vi "SRI8610C-ProcessSRILogFile.vi"(8 "error in":errorcluster) -> (0 "error out":errorcluster, 1 "Butane % Array":string[](array[string]), 2 "GC Full Data Channels":T1[](array[typedef]), 4 "Formatted Data Output":string[][](array[string]), 6 "Raw Data":string)   [LabVIEW 2020, in "SRI8610C-GasChromatograph.lvlib"]
uses:
  SRI8610C-GasChromatograph.lvlib
  Controls/SRI8610C-DataClusterV2.ctl
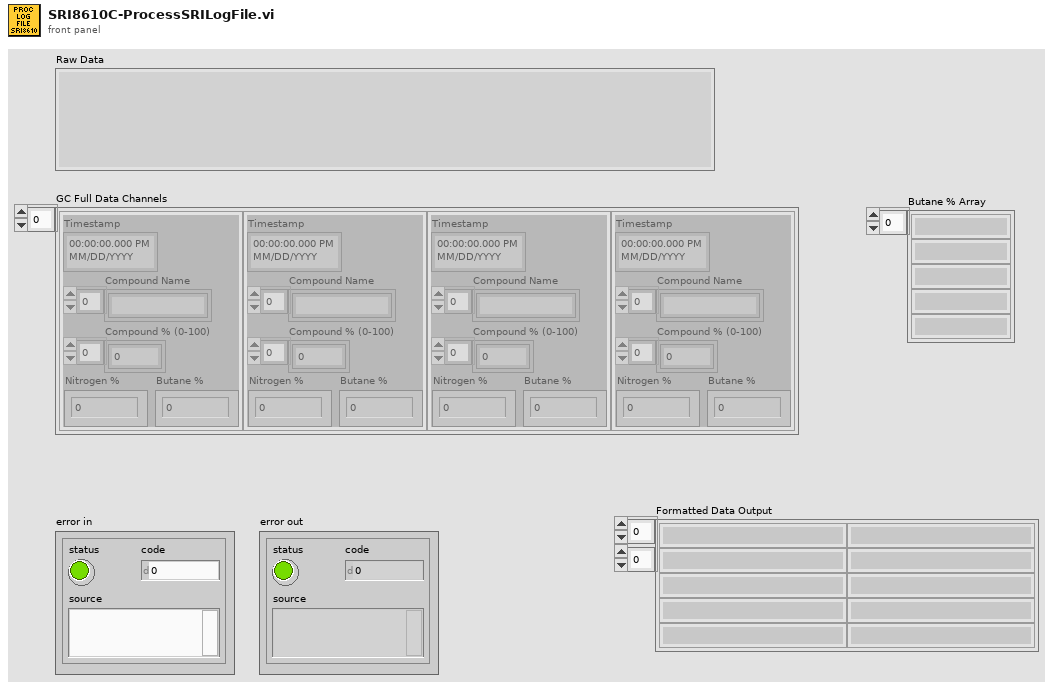
[diagram p1: front panel]
types:
  T1 = typedef "SRI8610C-DataClusterV2.ctl" = cluster{"Timestamp":timestamp, "Compound Name":string[], "Compound % (0-100)":dbl[], "Nitrogen %":dbl, "Butane %":dbl}
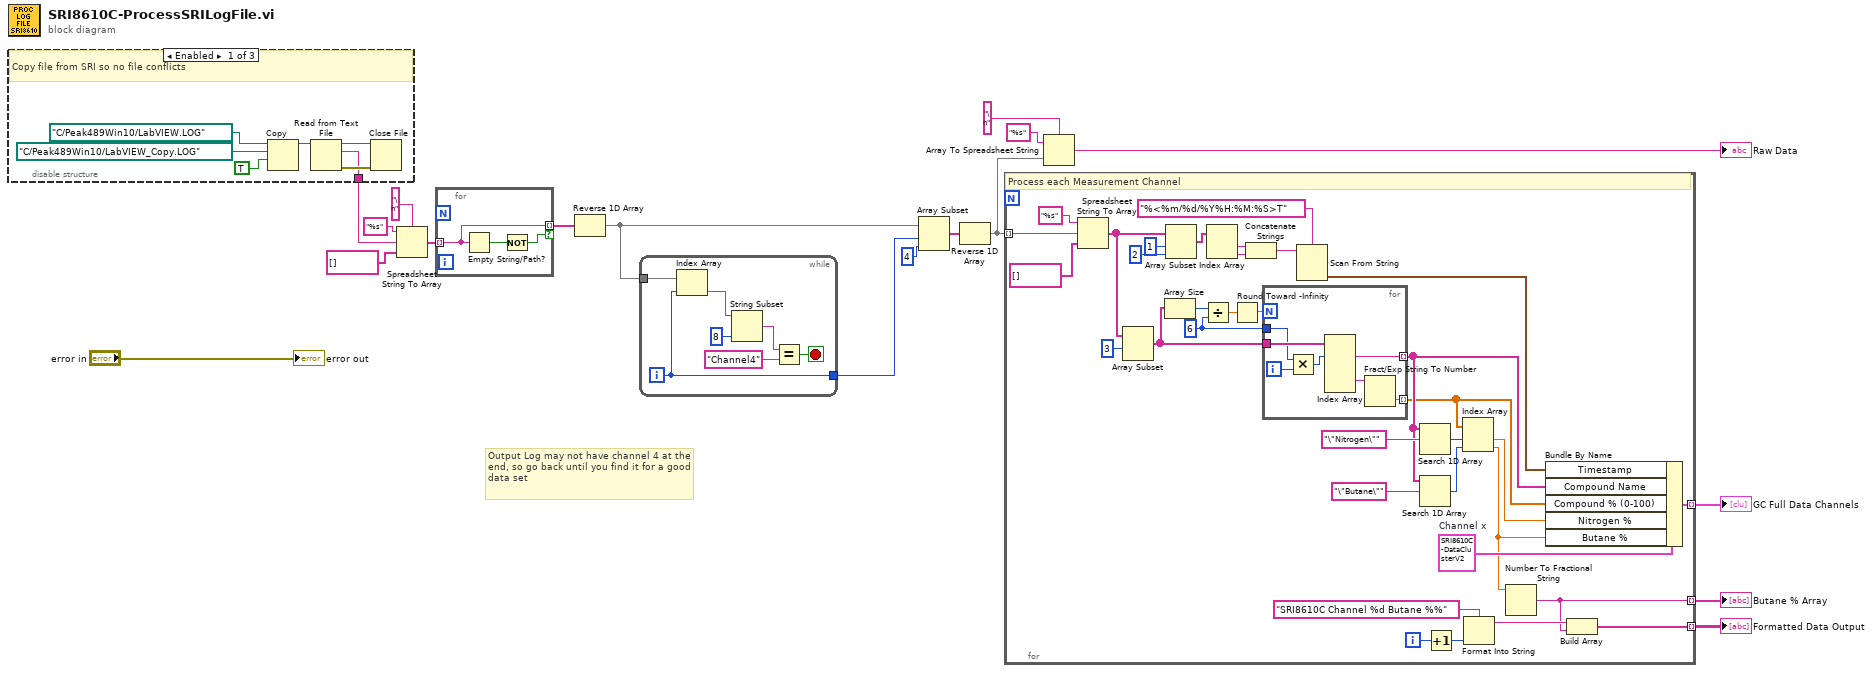
[diagram p0: block diagram]
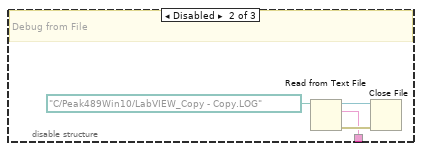
[diagram p2: hidden frame]
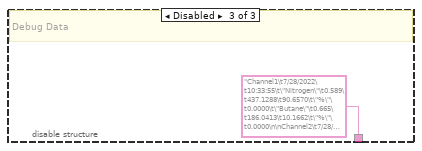
[diagram p3: hidden frame]
diagram:
  # "Output Log may not have channel 4 at the end, so go back until you find it for a good data set"
  n1 = disable-structure shown="Enabled" {
    disable-tunnel: [w23 w27 "﻿Channel1\t7/28/2022\t10:33:55\t\"Nitrogen\"\t0.589\t437.1288\t90.6570\t\"%\"\t0.0000\t\"Butane\"\t0.665\t186.0413\t10.1662\t\"%\"\t0.0000\n\nChannel2\t7/28/2022\t10:33:55\t\"Nitrogen\"\t0.607\t445.1454\t90.2536\t\"\"\t0.0000\t\"Butane\"\t0.689\t390.9493\t10.1440\t\"\"\t0.0000\n\nChannel3\t7/28/2022\t10:33:55\t\"Nitrogen\"\t0.637\t505.2661\t92.9726\t\"\"\t0.0000\t\"Butane\"\t0.717\t171.6732\t10.2985\t\"\"\t0.0000\n\nChannel4\t7/28/2022\t10:33:55\t\"Nitrogen\"\t0.679\t389.7807\t95.5677\t\"\"\t0.0000\t\"Butane\"\t0.772\t106.6082\t11.6693\t\"\"\t0.0000\n\nChannel1\t7/28/2022\t10:35:54\t\"Nitrogen\"\t0.588\t438.0254\t90.8429\t\"%\"\t0.0000\t\"Butane\"\t0.665\t185.9064\t10.1589\t\"%\"\t0.0000\n\nChannel2\t7/28/2022\t10:35:54\t\"Nitrogen\"\t0.609\t453.2789\t91.9027\t\"\"\t0.0000\t\"Butane\"\t0.690\t394.7194\t10.2418\t\"\"\t0.0000\n\nChannel3\t7/28/2022\t10:35:54\t\"Nitrogen\"\t0.633\t490.8435\t90.3187\t\"\"\t0.0000\t\"Butane\"\t0.712\t174.8892\t10.4915\t\"\"\t0.0000\n\nChannel4\t7/28/2022\t10:35:54\t\"Nitrogen\"\t0.679\t389.1852\t89.8625\t\"\"\t0.0000\t\"Butane\"\t0.772\t107.9233\t10.1234\t\"\"\t0.0000\n\nChannel1\t7/28/2022\t10:40:11\t\"Nitrogen\"\t0.586\t442.3609\t91.7421\t\"%\"\t0.0000\t\"Butane\"\t0.659\t185.3135\t10.1265\t\"%\"\t0.0000\n\nChannel2\t7/28/2022\t10:40:11\t\"Nitrogen\"\t0.611\t462.7982\t93.8327\t\"%\"\t0.0000\t\"Butane\"\t0.687\t396.2443\t10.2814\t\"%\"\t0.0000\n\nChannel3\t7/28/2022\t10:40:11\t\"Nitrogen\"\t0.631\t505.5395\t93.0229\t\"%\"\t0.0000\t\"Butane\"\t0.706\t177.1639\t10.6279\t\"%\"\t0.0000\n\nChannel4\t7/28/2022\t10:40:11\t\"Nitrogen\"\t0.678\t402.8086\t93.0081\t\"%\"\t0.0000\t\"Butane\"\t0.767\t110.6454\t10.3787\t\"%\"\t0.0000\n\nChannel1\t7/28/2022\t10:44:51\t\"Nitrogen\"\t0.592\t454.8368\t94.3295\t\"%\"\t0.0000\t\"Butane\"\t0.665\t185.1562\t10.1179\t\"%\"\t0.0000\n\nChannel2\t7/28/2022\t10:44:51\t\"Nitrogen\"\t0.613\t457.2752\t92.7129\t\"%\"\t0.0000\t\"Butane\"\t0.690\t384.0125\t9.9640\t\"%\"\t0.0000\n\nChannel3\t7/28/2022\t10:44:51\t\"Nitrogen\"\t0.634\t502.7721\t92.5136\t\"%\"\t0.0000\t\"Butane\"\t0.710\t172.8281\t10.3678\t\"%\"\t0.0000\n\nChannel4\t7/28/2022\t10:44:51\t\"Nitrogen\"\t0.685\t405.5581\t93.6430\t\"%\"\t0.0000\t\"Butane\"\t0.775\t105.0121\t9.8503\t\"%\"\t0.0000\n\nChannel1\t7/28/2022\t10:47:15\t\"Nitrogen\"\t0.593\t461.1496\t95.6387\t\"%\"\t0.0000\t\"Butane\"\t0.665\t206.6067\t11.2900\t\"%\"\t0.0000\n\nChannel2\t7/28/2022\t10:47:15\t\"Nitrogen\"\t0.615\t458.1744\t92.8952\t\"%\"\t0.0000\t\"Butane\"\t0.690\t392.6961\t10.1893\t\"%\"\t0.0000\n\nChannel3\t7/28/2022\t10:47:15\t\"Nitrogen\"\t0.640\t504.4086\t92.8148\t\"%\"\t0.0000\t\"Butane\"\t0.715\t175.3140\t10.5170\t\"%\"\t0.0000\n\nChannel4\t7/28/2022\t10:47:15\t\"Nitrogen\"\t0.690\t406.4146\t93.8407\t\"%\"\t0.0000\t\"Butane\"\t0.780\t108.7333\t10.1993\t\"%\"\t0.0000\n\nChannel1\t7/28/2022\t10:48:41\t\"Nitrogen\"\t0.589\t456.0841\t94.5882\t\"%\"\t0.0000\t\"Butane\"\t0.661\t187.6069\t10.2518\t\"%\"\t0.0000\n\nChannel2\t7/28/2022\t10:48:41\t\"Nitrogen\"\t0.610\t458.9680\t93.0561\t\"%\"\t0.0000\t\"Butane\"\t0.685\t389.9955\t10.1192\t\"%\"\t0.0000\n\nChannel3\t7/28/2022\t10:48:41\t\"Nitrogen\"\t0.634\t523.7252\t96.3692\t\"%\"\t0.0000\t\"Butane\"\t0.709\t173.7021\t10.4203\t\"%\"\t0.0000\n\nChannel4\t7/28/2022\t10:48:41\t\"Nitrogen\"\t0.680\t403.0654\t93.0674\t\"%\"\t0.0000\t\"Butane\"\t0.770\t106.7198\t10.0105\t\"%\"\t0.0000\n\nChannel1\t7/28/2022\t10:49:41\t\"Nitrogen\"\t0.586\t452.1232\t93.7667\t\"%\"\t0.0000\t\"Butane\"\t0.658\t193.7669\t10.5884\t\"%\"\t0.0000\n\nChannel2\t7/28/2022\t10:49:41\t\"Nitrogen\"\t0.610\t449.0700\t91.0493\t\"%\"\t0.0000\t\"Butane\"\t0.686\t387.2711\t10.0485\t\"%\"\t0.0000\n\nChannel3\t7/28/2022\t10:49:41\t\"Nitrogen\"\t0.634\t505.1364\t92.9487\t\"%\"\t0.0000\t\"Butane\"\t0.709\t173.6331\t10.4161\t\"%\"\t0.0000\n\nChannel4\t7/28/2022\t10:49:41\t\"Nitrogen\"\t0.680\t404.8906\t93.4889\t\"%\"\t0.0000\t\"Butane\"\t0.770\t109.0485\t10.2289\t\"%\"\t0.0000\n\nChannel1\t7/28/2022\t10:50:41\t\"Nitrogen\"\t0.586\t443.3960\t91.9568\t\"%\"\t0.0000\t\"Butane\"\t0.663\t187.3666\t10.2387\t\"%\"\t0.0000\n\nChannel2\t7/28/2022\t10:50:41\t\"Nitrogen\"\t0.607\t443.3777\t89.8952\t\"%\"\t0.0000\t\"Butane\"\t0.688\t386.9407\t10.0400\t\"%\"\t0.0000\n\nChannel3\t7/28/2022\t10:50:41\t\"Nitrogen\"\t0.633\t495.6569\t91.2044\t\"%\"\t0.0000\t\"Butane\"\t0.711\t173.5282\t10.4098\t\"%\"\t0.0000\n\nChannel4\t7/28/2022\t10:50:41\t\"Nitrogen\"\t0.675\t387.4188\t89.4546\t\"%\"\t0.0000\t\"Butane\"\t0.768\t108.5366\t10.1809\t\"%\"\t0.0000\n\nChannel1\t7/28/2022\t10:51:41\t\"Nitrogen\"\t0.586\t443.9583\t92.0734\t\"%\"\t0.0000\t\"Butane\"\t0.663\t192.7158\t10.5310\t\"%\"\t0.0000\n\nChannel2\t7/28/2022\t10:51:41\t\"Nitrogen\"\t0.608\t448.7605\t90.9865\t\"%\"\t0.0000\t\"Butane\"\t0.689\t393.1967\t10.2023\t\"%\"\t0.0000\n\nChannel3\t7/28/2022\t10:51:41\t\"Nitrogen\"\t0.630\t486.5227\t89.5236\t\"%\"\t0.0000\t\"Butane\"\t0.708\t174.0483\t10.4410\t\"%\"\t0.0000\n\nChannel4\t7/28/2022\t10:51:41\t\"Nitrogen\"\t0.675\t388.9742\t89.8138\t\"%\"\t0.0000\t\"Butane\"\t0.769\t111.8752\t10.4940\t\"%\"\t0.0000\n\nChannel1\t7/28/2022\t10:52:41\t\"Nitrogen\"\t0.586\t441.9869\t91.6645\t\"%\"\t0.0000\t\"Butane\"\t0.662\t187.2055\t10.2299\t\"%\"\t0.0000\n\nChannel2\t7/28/2022\t10:52:41\t\"Nitrogen\"\t0.604\t446.4374\t90.5155\t\"%\"\t0.0000\t\"Butane\"\t0.684\t389.8585\t10.1157\t\"%\"\t0.0000\n\nChannel3\t7/28/2022\t10:52:41\t\"Nitrogen\"\t0.632\t498.5583\t91.7383\t\"%\"\t0.0000\t\"Butane\"\t0.710\t173.4587\t10.4057\t\"%\"\t0.0000\n\nChannel4\t7/28/2022\t10:52:41\t\"Nitrogen\"\t0.675\t401.6506\t92.7407\t\"%\"\t0.0000\t\"Butane\"\t0.769\t113.5704\t10.6531\t\"%\"\t0.0000\n\nChannel1\t7/28/2022\t10:53:41\t\"Nitrogen\"\t0.589\t441.0544\t91.4711\t\"%\"\t0.0000\t\"Butane\"\t0.665\t190.6689\t10.4191\t\"%\"\t0.0000\n\nChannel2\t7/28/2022\t10:53:41\t\"Nitrogen\"\t0.603\t440.6179\t89.3356\t\"%\"\t0.0000\t\"Butane\"\t0.684\t387.5953\t10.0569\t\"%\"\t0.0000\n\nChannel3\t7/28/2022\t10:53:41\t\"Nitrogen\"\t0.634\t491.4375\t90.4280\t\"%\"\t0.0000\t\"Butane\"\t0.712\t173.4105\t10.4028\t\"%\"\t0.0000\n\nChannel4\t7/28/2022\t10:53:41\t\"Nitrogen\"\t0.675\t389.1500\t89.8544\t\"%\"\t0.0000\t\"Butane\"\t0.767\t115.9844\t10.8795\t\"%\"\t0.0000\n\nChannel1\t7/28/2022\t10:54:41\t\"Nitrogen\"\t0.584\t431.0600\t89.3984\t\"%\"\t0.0000\t\"Butane\"\t0.660\t186.8141\t10.2085\t\"%\"\t0.0000\n\nChannel2\t7/28/2022\t10:54:41\t\"Nitrogen\"\t0.610\t444.6270\t90.1485\t\"%\"\t0.0000\t\"Butane\"\t0.690\t393.6837\t10.2149\t\"%\"\t0.0000\n\nChannel3\t7/28/2022\t10:54:41\t\"Nitrogen\"\t0.632\t489.1760\t90.0119\t\"%\"\t0.0000\t\"Butane\"\t0.710\t174.7053\t10.4804\t\"%\"\t0.0000\n\nChannel4\t7/28/2022\t10:54:41\t\"Nitrogen\"\t0.677\t394.4412\t91.0761\t\"%\"\t0.0000\t\"Butane\"\t0.770\t117.7810\t11.0480\t\"%\"\t0.0000\n\nChannel1\t7/28/2022\t10:55:41\t\"Nitrogen\"\t0.580\t427.2364\t88.6054\t\"%\"\t0.0000\t\"Butane\"\t0.656\t187.9701\t10.2716\t\"%\"\t0.0000\n\nChannel2\t7/28/2022\t10:55:41\t\"Nitrogen\"\t0.609\t446.4921\t90.5266\t\"%\"\t0.0000\t\"Butane\"\t0.690\t389.7151\t10.1119\t\"%\"\t0.0000\n\nChannel3\t7/28/2022\t10:55:41\t\"Nitrogen\"\t0.628\t488.3736\t89.8642\t\"%\"\t0.0000\t\"Butane\"\t0.706\t174.7363\t10.4823\t\"%\"\t0.0000\n\nChannel4\t7/28/2022\t10:55:41\t\"Nitrogen\"\t0.674\t389.1800\t89.8613\t\"%\"\t0.0000\t\"Butane\"\t0.767\t121.1649\t11.3654\t\"%\"\t0.0000\n\nChannel1\t7/28/2022\t10:56:41\t\"Nitrogen\"\t0.585\t435.3329\t90.2846\t\"%\"\t0.0000\t\"Butane\"\t0.661\t194.0965\t10.6064\t\"%\"\t0.0000\n\nChannel2\t7/28/2022\t10:56:41\t\"Nitrogen\"\t0.607\t442.1884\t89.6541\t\"%\"\t0.0000\t\"Butane\"\t0.688\t389.5965\t10.1089\t\"%\"\t0.0000\n\nChannel3\t7/28/2022\t10:56:41\t\"Nitrogen\"\t0.632\t486.6515\t89.5473\t\"%\"\t0.0000\t\"Butane\"\t0.710\t174.0195\t10.4393\t\"%\"\t0.0000\n\nChannel4\t7/28/2022\t10:56:41\t\"Nitrogen\"\t0.677\t386.0838\t89.1464\t\"%\"\t0.0000\t\"Butane\"\t0.770\t121.0938\t11.3588\t\"%\"\t0.0000\n\nChannel1\t7/28/2022\t11:07:10\t\"Nitrogen\"\t0.589\t443.9774\t92.0773\t\"%\"\t0.0000\t\"Butane\"\t0.665\t192.2419\t10.5051\t\"%\"\t0.0000\n\nChannel2\t7/28/2022\t11:07:10\t\"Nitrogen\"\t0.610\t446.4577\t90.5196\t\"%\"\t0.0000\t\"Butane\"\t0.691\t396.5257\t10.2887\t\"%\"\t0.0000\n\nChannel3\t7/28/2022\t11:07:10\t\"Nitrogen\"\t0.635\t496.3736\t91.3363\t\"%\"\t0.0000\t\"Butane\"\t0.712\t178.6805\t10.7189\t\"%\"\t0.0000\n\nChannel4\t7/28/2022\t11:07:10\t\"Nitrogen\"\t0.680\t393.4634\t90.8503\t\"%\"\t0.0000\t\"Butane\"\t0.772\t128.0492\t12.0112\t\"%\"\t0.0000\n\nChannel1\t7/28/2022\t11:08:10\t\"Nitrogen\"\t0.582\t431.7955\t89.5509\t\"%\"\t0.0000\t\"Butane\"\t0.659\t189.6235\t10.3620\t\"%\"\t0.0000\n\nChannel2\t7/28/2022\t11:08:10\t\"Nitrogen\"\t0.608\t448.0522\t90.8429\t\"%\"\t0.0000\t\"Butane\"\t0.689\t393.3569\t10.2064\t\"%\"\t0.0000\n\nChannel3\t7/28/2022\t11:08:10\t\"Nitrogen\"\t0.630\t498.1358\t91.6605\t\"%\"\t0.0000\t\"Butane\"\t0.708\t177.7221\t10.6614\t\"%\"\t0.0000\n\nChannel4\t7/28/2022\t11:08:10\t\"Nitrogen\"\t0.673\t390.2655\t90.1120\t\"%\"\t0.0000\t\"Butane\"\t0.765\t127.8608\t11.9935\t\"%\"\t0.0000\n\nChannel1\t7/28/2022\t11:09:10\t\"Nitrogen\"\t0.590\t439.6186\t91.1734\t\"%\"\t0.0000\t\"Butane\"\t0.666\t190.6637\t10.4188\t\"%\"\t0.0000\n\nChannel2\t7/28/2022\t11:09:10\t\"Nitrogen\"\t0.600\t436.6578\t88.5327\t\"%\"\t0.0000\t\"Butane\"\t0.680\t393.9048\t10.2206\t\"%\"\t0.0000\n\nChannel3\t7/28/2022\t11:09:10\t\"Nitrogen\"\t0.629\t489.8129\t90.1291\t\"%\"\t0.0000\t\"Butane\"\t0.707\t174.9043\t10.4924\t\"%\"\t0.0000\n\nChannel4\t7/28/2022\t11:09:10\t\"Nitrogen\"\t0.674\t394.6286\t91.1194\t\"%\"\t0.0000\t\"Butane\"\t0.765\t131.7629\t12.3595\t\"%\"\t0.0000\n\nChannel1\t7/28/2022\t11:10:10\t\"Nitrogen\"\t0.585\t436.7208\t90.5724\t\"%\"\t0.0000\t\"Butane\"\t0.662\t189.3785\t10.3486\t\"%\"\t0.0000\n\nChannel2\t7/28/2022\t11:10:10\t\"Nitrogen\"\t0.606\t441.9639\t89.6085\t\"%\"\t0.0000\t\"Butane\"\t0.687\t393.4348\t10.2085\t\"%\"\t0.0000\n\nChannel3\t7/28/2022\t11:10:10\t\"Nitrogen\"\t0.633\t492.0724\t90.5448\t\"%\"\t0.0000\t\"Butane\"\t0.711\t176.6468\t10.5969\t\"%\"\t0.0000\n\nChannel4\t7/28/2022\t11:10:10\t\"Nitrogen\"\t0.675\t392.5132\t90.6309\t\"%\"\t0.0000\t\"Butane\"\t0.767\t132.6564\t12.4434\t\"%\"\t0.0000\n\nChannel1\t7/28/2022\t11:11:10\t\"Nitrogen\"\t0.592\t447.0001\t92.7042\t\"%\"\t0.0000\t\"Butane\"\t0.670\t189.5167\t10.3562\t\"%\"\t0.0000\n\nChannel2\t7/28/2022\t11:11:10\t\"Nitrogen\"\t0.605\t444.0000\t90.0213\t\"%\"\t0.0000\t\"Butane\"\t0.685\t392.2206\t10.1769\t\"%\"\t0.0000\n\nChannel3\t7/28/2022\t11:11:10\t\"Nitrogen\"\t0.628\t487.5794\t89.7181\t\"%\"\t0.0000\t\"Butane\"\t0.705\t178.4825\t10.7070\t\"%\"\t0.0000\n\nChannel4\t7/28/2022\t11:11:10\t\"Nitrogen\"\t0.674\t396.2380\t91.4910\t\"%\"\t0.0000\t\"Butane\"\t0.766\t131.5262\t12.3373\t\"%\"\t0.0000\n\n" ("text")] -> w15
    frame Enabled {
      # "Copy file from SRI so no file conflicts"
      n2 = Copy(9:TRUE ("overwrite (F)"), 10:path "C:/Peak489Win10/LabVIEW_Copy.LOG" ("target path (use dialog)"), 11:path "C:/Peak489Win10/LabVIEW.LOG" ("file (use dialog)")) -> (3:w19:path)  [unwired: 2 in, 2 out]
      n3 = Read from Text File(file (use dialog)=w19) -> (refnum out=w25:refnum<file>, text=w23:string, error out=w24:errorcluster)  [unwired: 3 in, 1 out]
      n4 = Close File(refnum=w25, error in=w24) -> ()  [unwired: 2 out]
    }
    frame Disabled {
      # "Debug from File"
      n5 = Read from Text File(file (use dialog)=path "C:/Peak489Win10/LabVIEW_Copy - Copy.LOG") -> (refnum out=w29:refnum<file>, text=w27:string, error out=w28:errorcluster)  [unwired: 3 in, 1 out]
      n6 = Close File(refnum=w29, error in=w28) -> ()  [unwired: 2 out]
    }
    frame Disabled {
      # "Debug Data"
    }
  }
  n7 = Spreadsheet String To Array(delimiter (Tab)="\n", format string="%s", spreadsheet string=w15, array type (2D Dbl)=string[] []) -> (array=w11:string[])
  n8 = for {
    tunnel: w11 -> [w33] mode=indexing
    tunnel: [w33] -> w10 mode=indexing if=w31
    n9 = Empty String/Path?(string/path=w33) -> (empty?=w32:bool)
    n10 = Not(x=w32) -> (.not. x?=w31:bool)
  }
  n11 = Reverse 1D Array(array=w10) -> (reversed array=w1:string[])
  n12 = while {
    tunnel: [w40] -> w2
    tunnel: w1 -> [w39]
    i -> [w40]
    stop <- w34 stop-if-true
    n13 = Index Array(array=w39, index=w40) -> (element=w38:string)
    n14 = String Subset(string=w38, length (rest)=8 ("length (rest)")) -> (substring=w36:string)  [unwired: 1 in]
    n15 = Equal?(x=w36, y="Channel4") -> (x = y?=w34:bool)
  }
  n16 = Array Subset(array=w1, index=w2, length=4) -> (w8:string[])
  n17 = Reverse 1D Array(array=w8) -> (reversed array=w7:string[])
  n18 = for {
    tunnel: w7 -> [w74] mode=indexing
    tunnel: [w48] -> w18 mode=indexing
    tunnel: [w42] -> w4 mode=indexing
    tunnel: [w41] -> w3 mode=indexing
    i -> [w46]
    w57 = T1 {"Timestamp"=timestamp(0 s since 1904-01-01), "Compound Name"=[], "Compound % (0-100)"=[], "Nitrogen %"=0.0, "Butane %"=0.0}  # Channel x
    w58 = 6 ("y")
    # "Process each Measurement Channel"
    n19 = Spreadsheet String To Array(format string="%s", spreadsheet string=w74, array type (2D Dbl)=string[] []) -> (array=w64:string[])  [unwired: 1 in]
    n20 = Array Subset(array=w64, index=3) -> (w62:string[])  [unwired: 1 in]
    n21 = Array Size(array=w62) -> (size(s)=w61:i32)
    n22 = Array Subset(array=w64, index=1, length=2) -> (w69:string[])
    n23 = Divide(x=w61, y=w58) -> (x/y=w60:dbl)
    n24 = Index Array(array=w69) -> (element #1=w68:string, element #2=w67:string)  [unwired: 2 in]
    n25 = Round Toward -Infinity(1:w60) -> (0:w59:dbl)
    n26 = Concatenate Strings(w68, w67) -> (w66:string)
    n27 = for {
      N: w59 -> [_]
      tunnel: w62 -> [w79]
      tunnel: [w78] -> w53 mode=indexing
      tunnel: [w76] -> w50 mode=indexing
      tunnel: w58 -> [w75]
      i -> [w81]
      n28 = Multiply(x=w75, y=w81) -> (x*y=w80:i32)
      n29 = Index Array(array=w79, index #1=w80) -> (element #1=w78:string, element #4=w77:string)  [unwired: 4 in, 3 out]
      n30 = Fract/Exp String To Number(string=w77) -> (number=w76:dbl)  [unwired: 3 in, 1 out]
    }
    n31 = Scan From String(format string="%<%m/%d/%Y%H:%M:%S>T", input string=w66) -> (output 1=w56:timestamp)  [unwired: 3 in, 3 out]
    n32 = Search 1D Array(1D array=w53, element="\"Nitrogen\"") -> (index of element=w52:i32)  [unwired: 1 in]
    n33 = Search 1D Array(1D array=w53, element="\"Butane\"") -> (index of element=w51:i32)  [unwired: 1 in]
    n34 = Increment(x=w46) -> (x+1=w45:i32)
    n35 = Index Array(array=w50, index #1=w52, index #2=w51) -> (element #1=w49:dbl, element #2=w47:dbl)
    n36 = Format Into String(format string="SRI8610C Channel %d Butane %%", w45) -> (resulting string=w43:string)  [unwired: 2 in, 1 out]
    n37 = Number To Fractional String(number=w47) -> (F-format string=w41:string)  [unwired: 3 in]
    n38 = Bundle By Name(cluster=w57, "Timestamp"=w56, "Compound Name"=w53, "Compound % (0-100)"=w50, "Nitrogen %"=w49, "Butane %"=w47) -> (w48:T1)
    n39 = Build Array(w43, w41) -> (w42:string[])
  }
  "GC Full Data Channels" <- w18
  "Butane % Array" <- w3
  "Formatted Data Output" <- w4
  n40 = Array To Spreadsheet String(delimiter (Tab)="\n", array=w7, 3:"%s" ("format string")) -> (spreadsheet string=→"Raw Data":string)
  "error out" <- "error in"
